vi "initiatePartsTracking.vi"(8 "error in (no error)":errorcluster, 11 "reference in":refnum<class "Project Panels.lvclass">) -> (0 "error out":errorcluster, 2 "data":string[][](array[string]), 3 "reference out":refnum<class "Project Panels.lvclass">)   [LabVIEW 2015, in "Project Panels.lvclass"]
uses:
  Project Panels.lvclass
  SYS/PartsTracking Controller_class/PartsTracking Controller.lvclass
  APP/partsTracking_class/partsTracking.lvclass
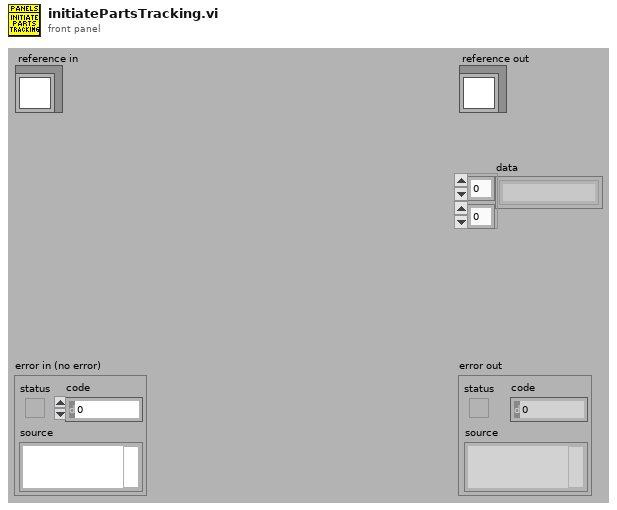
[diagram p1: front panel]
types:
  T1 = typedef "Project Panels.lvclass/ObjectAttributesRef.ctl" = refnum<data-value>
  T2 = typedef "Project Panels.lvclass/ObjectAttributes.ctl" = cluster{"MyAttribute":dbl, "device_controller_ref":refnum<class "Devices Controller.lvclass">, "file_controller_ref":refnum<class "File Controller.lvclass">, "item_controller_ref":refnum<class "Items Controller.lvclass">, "item_tables":cluster{"checkIN":string[][], "checkOUT":string[][], "storage":string[][]}, "quickbook_table":cluster{"notes":string[][]}, "notification_controller_ref":refnum<class "Notification Controller.lvclass">, "partstracking_controller_ref":refnum<class "PartsTracking Controller.lvclass">, "product_tables":cluster{"k4b2":string[][], "fitmate":string[][], "RMR":string[][], "CPET":string[][], "BP":string[][], "PP":string[][], "k5":string[][], "bb-pft":string[][]}, "rowsColour":u32[], "low_resolution?":bool}
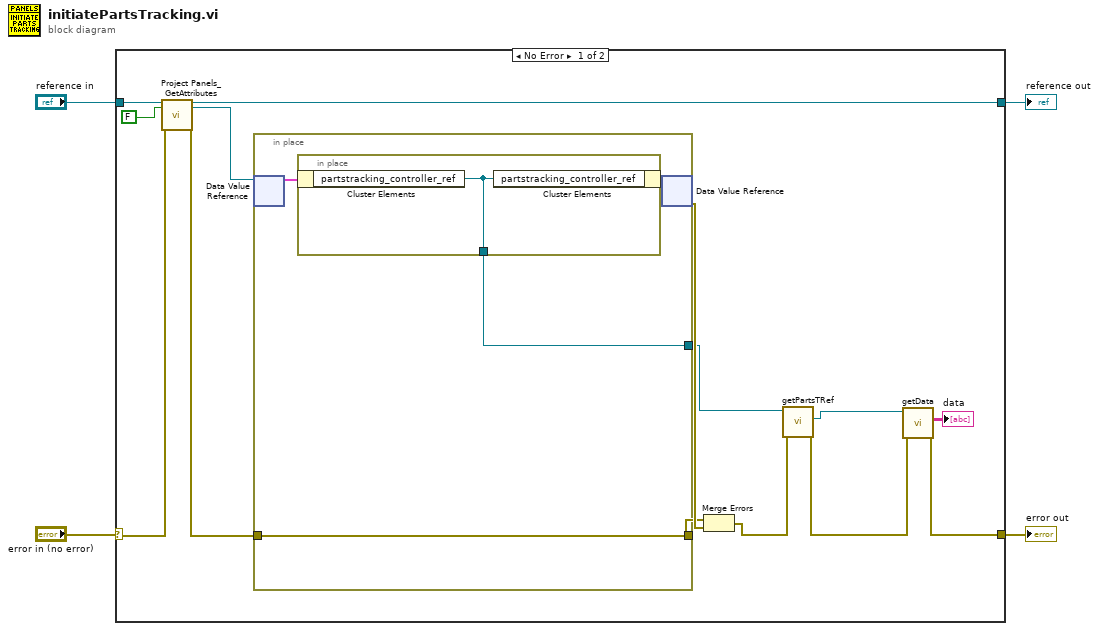
[diagram p0: block diagram]
diagram:
  n1 = case shown="No Error" "error in (no error)" {
    selector: "error in (no error)" -> [w14 w25]
    tunnel: [w6 w25] -> w3
    tunnel: [w12 w24] -> w1
    tunnel: "reference in" -> [w16 w24]
    frame No Error {
      n2 = call "Project Panels_GetAttributes.vi"("reference in"=w16, "return data? (T)"=FALSE, "error in (no error)"=w14) -> ("reference out"=w12:refnum<class "Project Panels.lvclass">, "attributes ref"=w11:T1, "error out"=w13:errorcluster)  [unwired: 13 in, 1 out]
      n3 = in-place {
        in-place-border: w13 -> [w20]
        in-place-border: [w20] -> w17
        in-place-border: [w19] -> w10
        n4 = in-place-dvr #1(w11) -> (w21:T2)  [unwired: 1 out]
        n5 = in-place {
          in-place-border: [w23] -> w19
          n6 = in-place-cluster #2(w21) -> ("partstracking_controller_ref"=w23:refnum<class "PartsTracking Controller.lvclass">)
          n7 = in-place-cluster #2("partstracking_controller_ref"=w23) -> (w22:T2)
        }
        n8 = in-place-dvr #1(w22) -> (w18:errorcluster)  [unwired: 1 out]
      }
      n9 = Merge Errors(w17, w18) -> (w9:errorcluster)
      n10 = call "getPartsTRef.vi"("error in (no error)"=w9, "reference in"=w10) -> ("error out"=w7:errorcluster, "partsTracking_ref"=w8:refnum<class "partsTracking.lvclass">)  [unwired: 7 in, 1 out]
      n11 = call "getData.vi"("error in (no error)"=w7, "reference in"=w8) -> ("error out"=w6:errorcluster, "data"=→"data":string[][])  [unwired: 7 in, 1 out]
    }
    frame Error {
    }
  }
  "error out" <- w3
  "reference out" <- w1
